vi "Update State in Routing Channel.vi"(8 "error in (no error)":errorcluster, 9 "Routing State":T1, 10 "State":string, 11 "Channel Ref in":T3 format="%.0x") -> (0 "error out":errorcluster, 3 "Channel Ref out":T3=18446744073709551615 format="%.0x")   [LabVIEW 2017, in "Switch Scripting.lvlib"]
uses:
  Switch Scripting.lvlib
  <vilib>/NI Veristand/Custom Device API/Custom Device Item Ref.ctl
  Routing State.ctl
  Connection.ctl
  NationalInstruments.VeriStand.SystemDefinitionAPI
  Shared/Constants.vi
  Shared/Switch Shared.lvlib
  <vilib>/NI VeriStand/Custom Device API/Custom Device API.lvlib
panel:
  in  "update select":u16(ring) items=["name", "value", "description", "connection list", "all"]
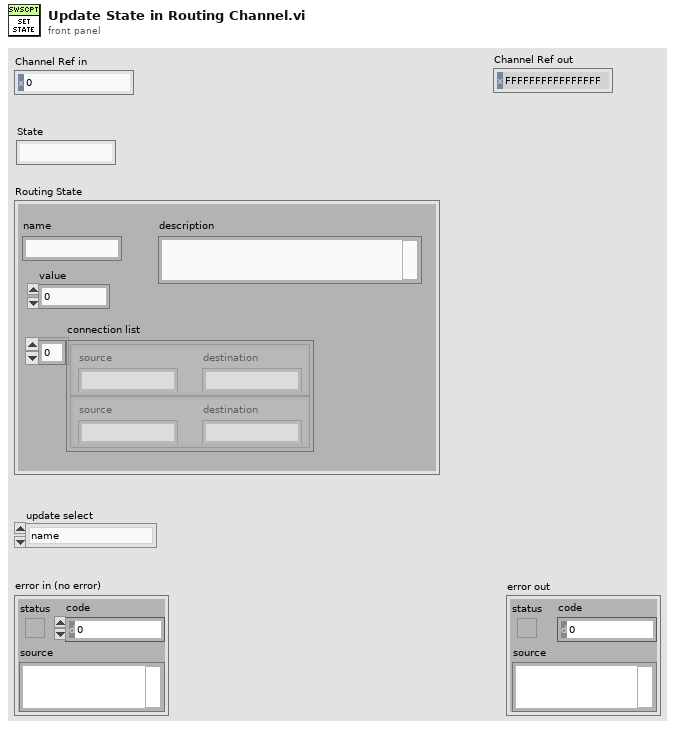
[diagram p1: front panel]
types:
  T1 = typedef "Switch Scripting.lvlib/Routing State.ctl" = cluster{"name":string, "description":string, "value":i32, "connection list":T2[]}
  T2 = typedef "Switch Scripting.lvlib/Connection.ctl" = cluster{"source":string, "destination":string}
  T3 = typedef "Custom Device API.lvlib/Custom Device Item Ref.ctl" = u64
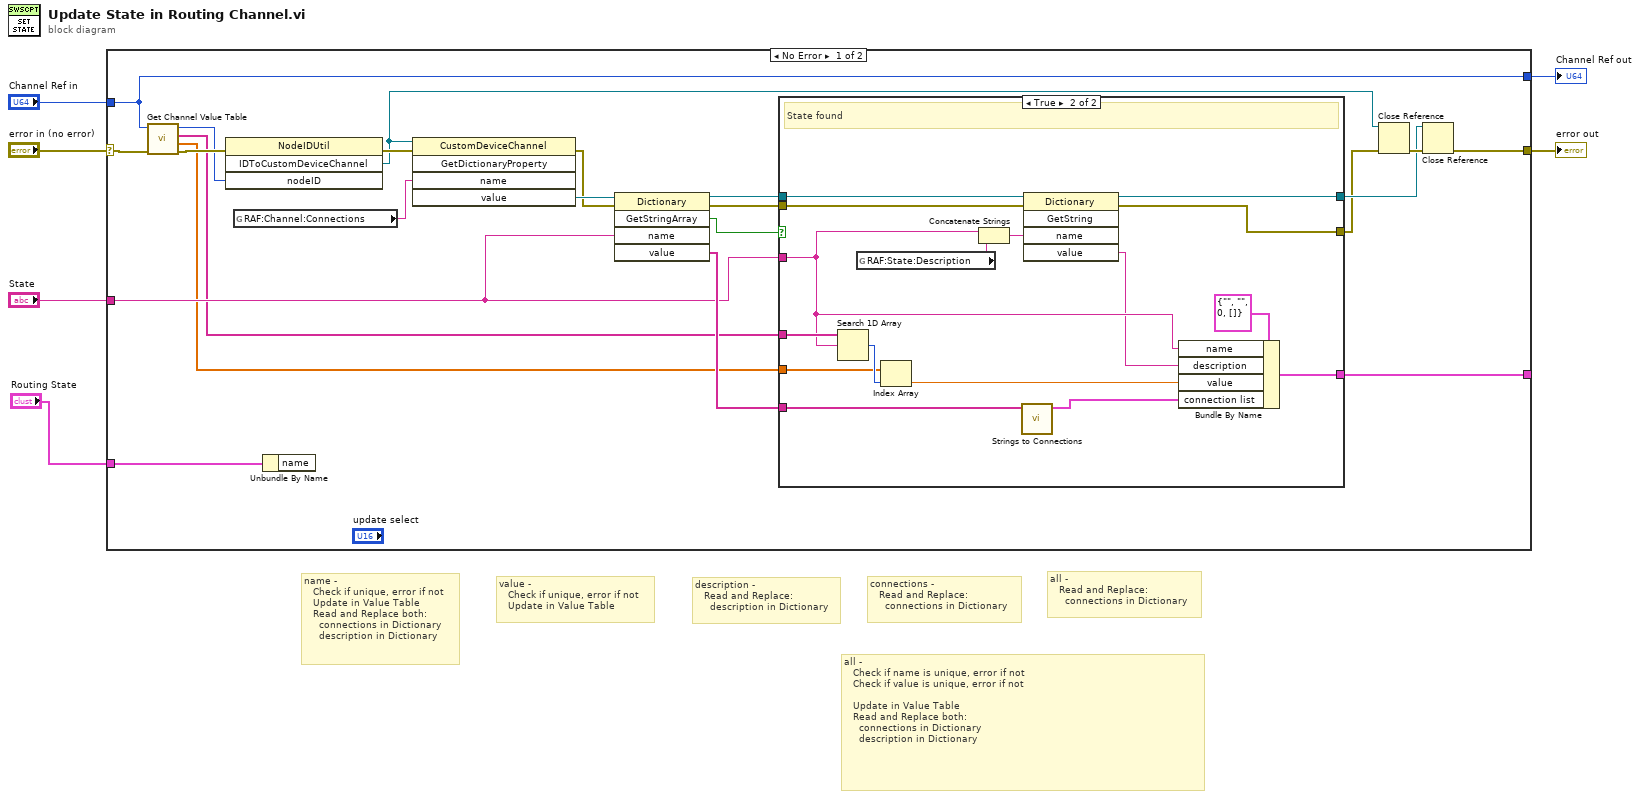
[diagram p0: block diagram]
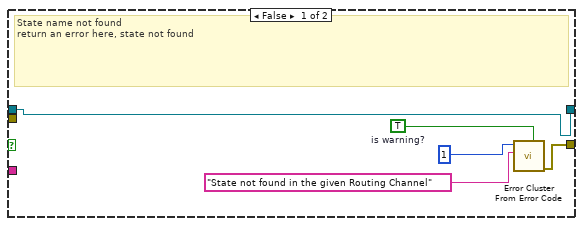
[diagram p2: hidden frame]
diagram:
  # "all -\n   Check if name is unique, error if not\n   Check if value is unique, error if not\n\n   Update in Value Table\n   Read and Replace both:\n     connections in Dictionary\n     description in Dictionary"
  # "all - \n   Read and Replace:\n     connections in Dictionary"
  # "connections - \n   Read and Replace:\n     connections in Dictionary"
  # "description - \n   Read and Replace:\n     description in Dictionary"
  # "value - \n   Check if unique, error if not\n   Update in Value Table"
  # "name - \n   Check if unique, error if not\n   Update in Value Table\n   Read and Replace both:\n     connections in Dictionary\n     description in Dictionary"
  n1 = case shown="No Error" "error in (no error)" {
    selector: "error in (no error)" -> [w14 w51]
    tunnel: [w28 w51] -> w5
    tunnel: "Channel Ref in" -> [w12 w50]
    tunnel: [w12 w50] -> w3
    tunnel: "State" -> [w15 _]
    tunnel: [w8 _] -> _
    tunnel: "Routing State" -> [w7 _]
    frame No Error {
      n2 = call "Get Channel Value Table.vi"("error in (no error)"=w14, "Channel Ref in"=w12) -> ("error out"=w13:errorcluster, "Values"=w9:dbl[], "States"=w10:string[], "Channel Ref out"=w11:T3)  [unwired: 6 in]
      n3 = invoke class="NodeIDUtil" method="IDToCustomDeviceChannel"(error in=w13, "nodeID"=w11) -> (error out=w26:errorcluster, "IDToCustomDeviceChannel"=w16:refnum<k24>)  [unwired: 2 in, 2 out]
      n4 = global read "Constants.vi" "RAF:Channel:Connections"() -> (w17:string)
      n5 = Unbundle By Name(w7) -> ()  [unwired: 1 out]
      n6 = invoke class="CustomDeviceChannel" method="GetDictionaryProperty"(reference=w16, error in=w26, "name"=w17) -> (error out=w23:errorcluster, "value"=w24:refnum<k24>)  [unwired: 2 in, 3 out]
      n7 = invoke class="Dictionary" method="GetStringArray"(reference=w24, error in=w23, "name"=w15) -> (reference out=w20:refnum<k24>, error out=w21:errorcluster, "GetStringArray"=w22:bool, "value"=w25:string[])  [unwired: 2 in, 1 out]
      n8 = case shown="True" w22 {
        tunnel: w25 -> [_ w37]
        tunnel: w21 -> [_ w39]
        tunnel: [w30 w40] -> w18
        tunnel: w20 -> [w29 w45]
        tunnel: [w29 w41] -> w19
        tunnel: w15 -> [_ w35]
        tunnel: w10 -> [_ w44]
        tunnel: w9 -> [_ w43]
        tunnel: [_ w38] -> w8
        frame False {
          w32 = TRUE  # is warning?
          # "State name not found\nreturn an error here, state not found"
          n9 = call <vilib>:"Error Cluster From Error Code.vi"("is warning? (False)"=w32, "error message (\"\")"="State not found in the given Routing Channel" ("error message (\"\")"), "error code (0)"=1) -> ("error out"=w30:errorcluster)  [unwired: 6 in]
        }
        frame True {
          # "State found"
          n10 = Search 1D Array(1D array=w44, element=w35) -> (index of element=w48:i32)  [unwired: 1 in]
          n11 = global read "Constants.vi" "RAF:State:Description"() -> (w47:string)
          n12 = Index Array(array=w43, index=w48) -> (element=w42:dbl)
          n13 = Concatenate Strings(w35, w47) -> (w46:string)
          n14 = call "Strings to Connections.vi"("connection strings"=w37) -> ("connection list"=w36:T2[])  [unwired: 10 in]
          n15 = invoke class="Dictionary" method="GetString"(reference=w45, error in=w39, "name"=w46) -> (reference out=w41:refnum<k24>, error out=w40:errorcluster, "value"=w34:string)  [unwired: 2 in, 2 out]
          n16 = Bundle By Name(cluster=T1 {"name"="", "description"="", "value"=0, "connection list"=[]} ("Routing State"), "name"=w35, "description"=w34, "value"=w42, "connection list"=w36) -> (w38:T1)
        }
      }
      n17 = Close Reference(reference=w16, error in (no error)=w18) -> (error out=w27:errorcluster)
      n18 = Close Reference(reference=w19, error in (no error)=w27) -> (error out=w28:errorcluster)
    }
    frame Error {
    }
  }
  "Channel Ref out" <- w3
  "error out" <- w5
